vi "SelectionTypeExample.vi"() -> ()   [LabVIEW 2016]
doc: "Run the VI and look under the \"Selection Types\" menu item for a demo of the built in selection types.\n\nAuthored by Derek E. Trepanier\nsupport@mooregoodideas.com\nwww.mooregoodideas.com\n\nCopyright (c) 2012, Moore Good Ideas, Inc.\n\nAll rights reserved.\n\nRedistribution and use in source and binary forms, with or without modification, are permitted provided that the following conditions are met:\n\n * Redistributions of source code must retain the above copyright notice, this list of conditions and the following disclaimer.\n * Redistributions in binary form must reproduce the above copyright notice, this list of conditions and the following disclaimer in the documentation and/or other materials provided with the distribution.\n * Neither the name of Moore Good Ideas, Inc. nor the names of its contributors may be used to endorse or promote products derived from this software without specific prior written permission.\n\nTHIS SOFTWARE IS PROVIDED BY THE COPYRIGHT HOLDERS AND CONTRIBUTORS \"AS IS\" AND ANY EXPRESS OR IMPLIED WARRANTIES, INCLUDING, BUT NOT LIMITED TO, THE IMPLIED WARRANTIES OF MERCHANTABILITY AND FITNESS FOR A PARTICULAR PURPOSE ARE DISCLAIMED. IN NO EVENT SHALL THE COPYRIGHT OWNER OR CONTRIBUTORS BE LIABLE FOR ANY DIRECT, INDIRECT, INCIDENTAL, SPECIAL, EXEMPLARY, OR CONSEQUENTIAL DAMAGES (INCLUDING, BUT NOT LIMITED TO, PROCUREMENT OF SUBSTITUTE GOODS OR SERVICES; LOSS OF USE, DATA, OR PROFITS; OR BUSINESS INTERRUPTION) HOWEVER CAUSED AND ON ANY THEORY OF LIABILITY, WHETHER IN CONTRACT, STRICT LIABILITY, OR TORT (INCLUDING NEGLIGENCE OR OTHERWISE) ARISING IN ANY WAY OUT OF THE USE OF THIS SOFTWARE, EVEN IF ADVISED OF THE POSSIBILITY OF SUCH DAMAGE."
uses:
  <userlib>/_MGI/Menu Building/SelectionType/RadioSelection/MGI_RadioSelection.lvclass
  C:/Program Files (x86)/National Instruments/LabVIEW 2016/user.lib/_MGI/Menu Building/SelectionType/MGI_SelectionType.lvclass
  <userlib>/_MGI/Menu Building/SelectionType/ToggleText/MGI_ToggleText.lvclass
  <userlib>/_MGI/Menu Building/SelectionType/CheckmarkSelection/MGI_CheckmarkSelection.lvclass
  <userlib>/_MGI/Menu Building/MenuItem/MenuSeparatorItem/MGI_MenuSeparatorItem.lvclass
  C:/Program Files (x86)/National Instruments/LabVIEW 2016/user.lib/_MGI/Menu Building/MenuItem/MGI_MenuItem.lvclass
  <userlib>/_MGI/Menu Building/SelectionType/RadioSelection/RadioSelection.vi
  <userlib>/_MGI/Menu Building/SelectionType/ToggleText/ToggleText.vi
  <userlib>/_MGI/Menu Building/MenuItem/MenuItem.vi
  <userlib>/_MGI/Menu Building/MenuItem/Write Click By Default.vi
  <userlib>/_MGI/Menu Building/MenuItem/Write Sub-Menus.vi
  <userlib>/_MGI/Menu Building/SelectionType/SelectionType.vi
  <userlib>/_MGI/Menu Building/SelectionType/CheckmarkSelection/CheckmarkSelection.vi
  <userlib>/_MGI/Menu Building/MenuItem/MenuSeparatorItem/MenuSeparatorItem.vi
  <userlib>/_MGI/Menu Building/MenuTypes/Vi/VI.vi
  <userlib>/_MGI/Menu Building/MenuTypes/Vi/MGI_VI.lvclass
  <userlib>/_MGI/Menu Building/MenuItem/MGI_MenuItem.lvclass
  <userlib>/_MGI/Menu Building/SelectionType/MGI_SelectionType.lvclass
  <userlib>/_MGI/Menu Building/MenuTypes/MGI_Menu.lvclass
  <userlib>/_MGI/Menu Building/MenuItemStatusChange/MGI_MenuItemStatusChange.lvclass
panel:
  out "History":T1(array[cluster])
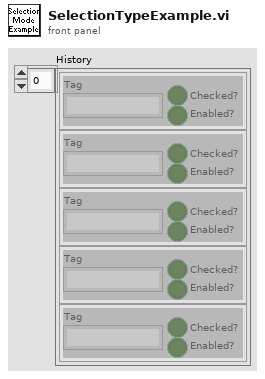
[diagram p1: front panel]
types:
  T1 = cluster{"Tag":string, "Checked?":bool, "Enabled?":bool}[]
  T2 = cluster{"Tag":string, "Checked?":bool, "Enabled?":bool}
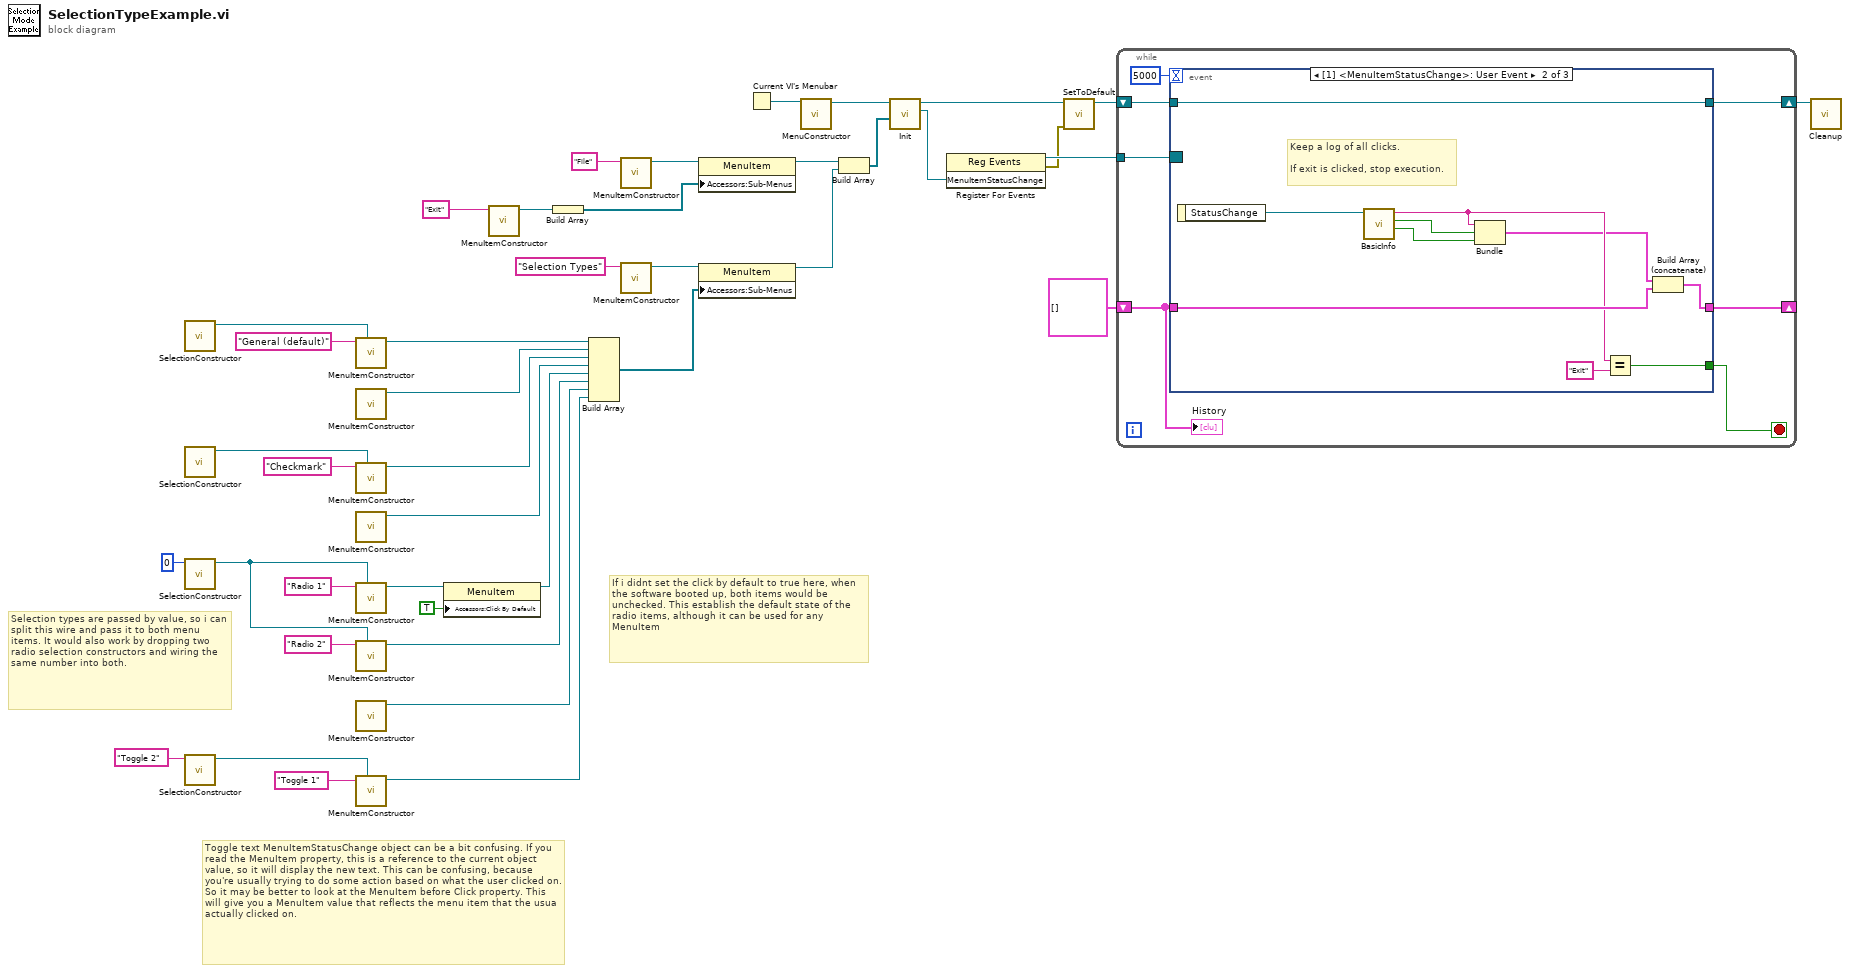
[diagram p0: block diagram]
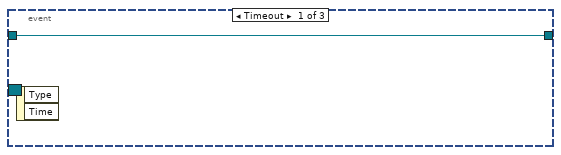
[diagram p2: hidden frame]
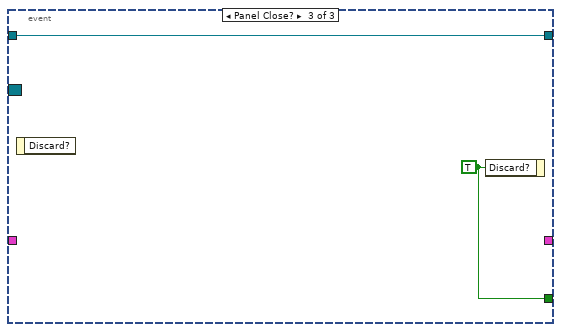
[diagram p3: hidden frame]
diagram:
  # "Toggle text MenuItemStatusChange object can be a bit confusing. If you read the MenuItem property, this is a reference to the current object value, so it will display the new text. This can be confusing, because you're usually trying to do some action based on what the user clicked on. So it may be better to look at the MenuItem before Click property. This will give you a MenuItem value that reflects the menu item that the usua actually clicked on."
  # "If i didnt set the click by default to true here, when the software booted up, both items would be unchecked. This establish the default state of the radio items, although it can be used for any MenuItem"
  # "Selection types are passed by value, so i can split this wire and pass it to both menu items. It would also work by dropping two radio selection constructors and wiring the same number into both."
  n1 = call-poly <userlib>:"SelectionConstructor.vi"() -> ("SelectionType out"=w41:refnum<class "MGI_SelectionType.lvclass">)  [unwired: 10 in, 1 out]
  n2 = call-poly <userlib>:"SelectionConstructor.vi"() -> ("CheckmarkSelection out"=w40:refnum<class "MGI_CheckmarkSelection.lvclass">)  [unwired: 10 in, 1 out]
  n3 = call-poly <userlib>:"SelectionConstructor.vi"("Group"=u8 0) -> ("RadioSelection out"=w38:refnum<class "MGI_RadioSelection.lvclass">)  [unwired: 9 in, 1 out]
  n4 = call-poly <userlib>:"SelectionConstructor.vi"("Secondary Text"="Toggle 2") -> ("ToggleText out"=w37:refnum<class "MGI_ToggleText.lvclass">)  [unwired: 9 in, 1 out]
  n5 = call-poly <userlib>:"MenuItemConstructor.vi"("Selection Type"=w41, "Text"="General (default)") -> ("MenuItem"=w35:refnum<data-value>)  [unwired: 8 in, 1 out]
  n6 = call-poly <userlib>:"MenuItemConstructor.vi"() -> ("MenuSeparatorItem"=w34:refnum<data-value>)  [unwired: 10 in, 1 out]
  n7 = call-poly <userlib>:"MenuItemConstructor.vi"("Selection Type"=w40, "Text"="Checkmark") -> ("MenuItem"=w33:refnum<data-value>)  [unwired: 8 in, 1 out]
  n8 = call-poly <userlib>:"MenuItemConstructor.vi"() -> ("MenuSeparatorItem"=w32:refnum<data-value>)  [unwired: 10 in, 1 out]
  n9 = call-poly <userlib>:"MenuItemConstructor.vi"("Selection Type"=w38, "Text"="Radio 1") -> ("MenuItem"=w31:refnum<data-value>)  [unwired: 8 in, 1 out]
  n10 = call-poly <userlib>:"MenuItemConstructor.vi"("Selection Type"=w38, "Text"="Radio 2") -> ("MenuItem"=w30:refnum<data-value>)  [unwired: 8 in, 1 out]
  n11 = call-poly <userlib>:"MenuItemConstructor.vi"() -> ("MenuSeparatorItem"=w29:refnum<data-value>)  [unwired: 10 in, 1 out]
  n12 = call-poly <userlib>:"MenuItemConstructor.vi"("Selection Type"=w37, "Text"="Toggle 1") -> ("MenuItem"=w28:refnum<data-value>)  [unwired: 8 in, 1 out]
  n13 = property class="MenuItem"(reference=w31, "Accessors:Click By Default"=TRUE ("Click By Default")) -> (reference out=w20:refnum<data-value>)  [unwired: 1 in, 1 out]
  n14 = call-poly <userlib>:"MenuItemConstructor.vi"("Text"="Exit") -> ("MenuItem"=w10:refnum<data-value>)  [unwired: 9 in, 1 out]
  n15 = Build Array(w10) -> (w8:refnum<data-value>[])
  n16 = Build Array(w35, w34, w33, w32, w20, w30, w29, w28) -> (w6:refnum<data-value>[])
  n17 = call-poly <userlib>:"MenuItemConstructor.vi"("Text"="File") -> ("MenuItem"=w9:refnum<data-value>)  [unwired: 9 in, 1 out]
  n18 = call-poly <userlib>:"MenuItemConstructor.vi"("Text"="Selection Types") -> ("MenuItem"=w7:refnum<data-value>)  [unwired: 9 in, 1 out]
  n19 = property class="MenuItem"(reference=w9, "Accessors:Sub-Menus"=w8) -> (reference out=w5:refnum<data-value>)  [unwired: 1 in, 1 out]
  n20 = property class="MenuItem"(reference=w7, "Accessors:Sub-Menus"=w6) -> (reference out=w4:refnum<data-value>)  [unwired: 1 in, 1 out]
  n21 = Current VI's Menubar() -> (w27:refnum<k9>)
  n22 = call-poly <userlib>:"MenuConstructor.vi"("menu reference"=w27) -> ("VI"=w26:refnum<class "MGI_VI.lvclass">)  [unwired: 9 in, 1 out]
  n23 = Build Array(w5, w4) -> (w3:refnum<data-value>[])
  n24 = call-dynamic "Init.vi"("Menu Items"=w3, "Menu in"=w26) -> ("MenuItemStatusChange"=w23:refnum<user-event>, "Menu out"=w22:refnum<class "MGI_VI.lvclass">)  [unwired: 7 in, 1 out]
  n25 = register-events(w23) -> (reference out=w24:refnum<event-registration>, error out=w2:errorcluster)  [unwired: 2 in]
  n26 = call-dynamic "SetToDefault.vi"("error in (no error)"=w2, "Menu in"=w22) -> ("Menu out"=w21:refnum<class "MGI_VI.lvclass">)  [unwired: 8 in, 1 out]
  n27 = while {
    tunnel: w24 -> [w48]
    shift-right: [w46] -> _
    shift-left: T1 [] -> [w44]
    shift-right: [w42] -> w25
    shift-left: w21 -> [w43]
    stop <- w47 stop-if-true
    n28 = event shown="[1] <MenuItemStatusChange>: User Event" {
      selector: w48 -> [_ _ _]
      dyn-events: _ -> [_ _ _]
      timeout: 5000 -> [_ _ _]
      tunnel: [_ w58 w61] -> w47
      tunnel: [_ w57 _] -> w46
      tunnel: w44 -> [_ w56 _]
      tunnel: w43 -> [w49 w55 w60]
      tunnel: [w49 w55 w60] -> w42
      event Timeout {
        n29 = event-data() -> ()  [unwired: 1 in, 2 out]
      }
      event User Event {
        # "Keep a log of all clicks.\n\nIf exit is clicked, stop execution."
        n30 = event-data() -> ("StatusChange"=w54:refnum<class "MGI_MenuItemStatusChange.lvclass">)  [unwired: 1 in]
        n31 = call <userlib>:"BasicInfo.vi"("MGI_MenuItemStatusChange in"=w54) -> ("Enabled?"=w51:bool, "Checked?"=w52:bool, "Tag"=w53:string)  [unwired: 7 in, 1 out]
        n32 = Bundle("Tag"=w53, "Checked?"=w52, "Enabled?"=w51) -> (w50:T2)  [unwired: 1 in]
        n33 = Equal?(x=w53, y="Exit") -> (x = y?=w58:bool)
        n34 = Build Array (concatenate)(w50, w56) -> (w57:T1)
      }
      event Panel Close? {
        w61 = TRUE ("Discard?")
        n35 = event-data() -> ()  [unwired: 1 in, 1 out]
        n36 = event-data("Discard?"=w61) -> ()  [unwired: 1 in, 1 out]
      }
    }
    "History" <- w44
  }
  n37 = call-dynamic "Cleanup.vi"("VI"=w25) -> ()  [unwired: 10 in, 1 out]
